vi "加标回收率计算.vi"(11 "参数":T1) -> (2 "加标后理论浓度":dbl, 3 "参数 out":T1)   [LabVIEW 2016, in "质控单元.lvlib"]
panel:
  out "V1(mL)":dbl
  out "R":dbl
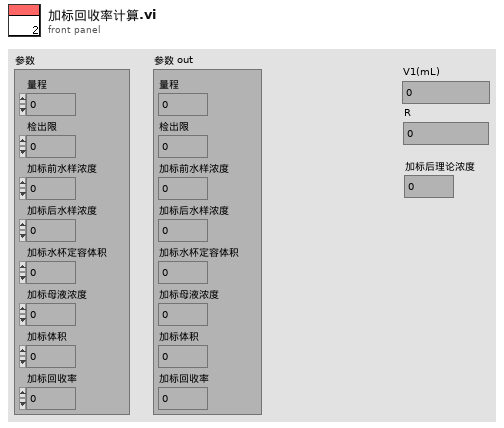
[diagram p1: front panel]
types:
  T1 = cluster{"量程":dbl, "检出限":dbl, "加标前水样浓度":dbl, "加标后水样浓度":dbl, "加标水杯定容体积":dbl, "加标母液浓度":dbl, "加标体积":dbl, "加标回收率":dbl}
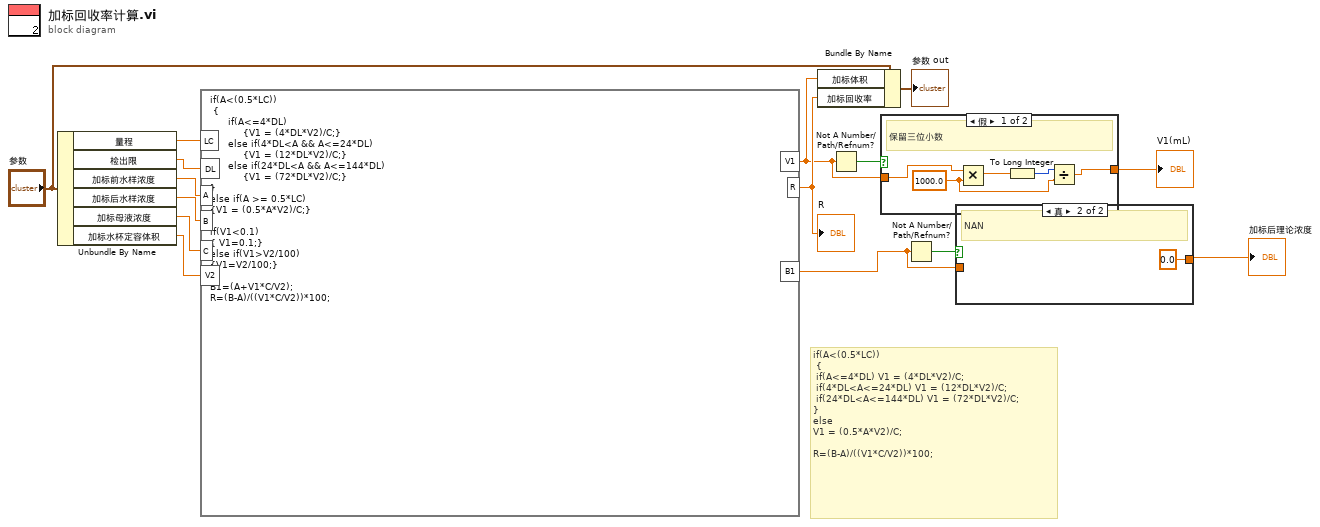
[diagram p0: block diagram]
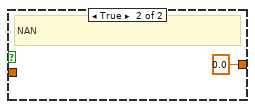
[diagram p3: hidden frame]
diagram:
  # "if(A<(0.5*LC))\n {\n if(A<=4*DL) V1 = (4*DL*V2)/C;\n if(4*DL<A<=24*DL) V1 = (12*DL*V2)/C;\n if(24*DL<A<=144*DL) V1 = (72*DL*V2)/C;\n}\nelse\nV1 = (0.5*A*V2)/C;\n\nR=(B-A)/((V1*C/V2))*100;"
  n1 = Unbundle By Name("参数") -> ("量程"=w12:dbl, "检出限"=w11:dbl, "加标前水样浓度"=w15:dbl, "加标后水样浓度"=w14:dbl, "加标母液浓度"=w13:dbl, "加标水杯定容体积"=w10:dbl)
  n2 = formula code="if(A<(0.5*LC))\n {\n      if(A<=4*DL) \n           {V1 = (4*DL*V2)/C;}\n      else if(4*DL<A && A<=24*DL) \n           {V1 = (12*DL*V2)/C;}\n      else if(24*DL<A && A<=144*DL) \n           {V1 = (72*DL*V2)/C;}\n}\nelse if(A >= 0.5*LC)\n{V1 = (0.5*A*V2)/C;}\n\nif(V1<0.1)\n{ V1=0.1;}\nelse if(V1>V2/100)\n{V1=V2/100;}\n\nB1=(A+V1*C/V2);\nR=(B-A)/((V1*C/V2))*100;"("A"=w15, "B"=w14, "C"=w13, "V2"=w10, "LC"=w12, "DL"=w11) -> ("R"=w8:dbl, "V1"=w5:dbl, "B1"=w2:dbl)
  "R" <- w8
  n3 = Bundle By Name(cluster="参数", "加标体积"=w5, "加标回收率"=w8) -> (→"参数 out":T1)
  n4 = Not A Number/Path/Refnum?(number/path/refnum=w5) -> (NaN/Path/Refnum?=w6:bool)
  n5 = case shown="假" w6 {
    tunnel: w5 -> [w20 _]
    tunnel: [w16 0.0] -> w4
    frame False {
      w17 = 1000.0 ("y")
      # "保留三位小数"
      n6 = Multiply(x=w20, y=w17) -> (x*y=w19:dbl)
      n7 = To Long Integer(number=w19) -> (32bit integer=w18:i32)
      n8 = Divide(x=w18, y=w17) -> (x/y=w16:dbl)
    }
    frame True {
      # "NAN"
    }
  }
  "V1(mL)" <- w4
  n9 = Not A Number/Path/Refnum?(number/path/refnum=w2) -> (NaN/Path/Refnum?=w3:bool)
  n10 = case shown="真" w3 {
    tunnel: w2 -> [w22 _]
    tunnel: [w22 0.0] -> w1
    frame False {
    }
    frame True {
      # "NAN"
    }
  }
  "加标后理论浓度" <- w1
